vi "Clock Divide by 2.vi"(11 "Reset?":bool) -> (3 "CLK/2":bool)   [LabVIEW 2012]
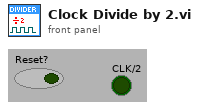
[diagram p1: front panel]
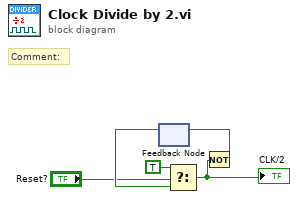
[diagram p0: block diagram]
diagram:
  # "Comment:"
  n1 = feedback #1() -> (w4:bool)  [unwired: 1 in]
  n2 = Select(t=TRUE, s="Reset?", f=w4) -> (s? t:f=w1:bool)
  "CLK/2" <- w1
  n3 = Not(x=w1) -> (.not. x?=w3:bool)
  n4 = feedback-in #1(w3) -> ()
